vi "Average Sectors.vi"   [LabVIEW 2013]
uses:
  Globals/Accumulated Sector Intensity.vi
  Globals/Sector Parameter Global.vi
  <vilib>/rvi/Memory/Memory_Emulation/nirvimemoryFastEmulationFpgaImpl.vi
  <instcachedir>/0/nirvimemoryFastEmulationFpgaImpl_5FBAB50466BC4C939F684F8805638BFC.lvgen/nirvimemoryFastEmulationFpgaImpl_5FBAB50466BC4C939F684F8805638BFC_006.vi
  <vilib>/rvi/DataTransferAndStorage/Container/Common/niFpgaContainerGetUniqueNameForEmu.vi
  <vilib>/rvi/Memory/Memory_Emulation/nirvimemoryFastEmulation.vi
  <vilib>/rvi/Memory/Memory_Emulation/nirvimemoryEmulation.vi
  <vilib>/rvi/FIFO/Fifo_Resource/nirvififoEmulationWriteFpgaImpl.vi
  <vilib>/rvi/DataTransferAndStorage/Container/XNode/niFpgaContainer.xnode
  <vilib>/rvi/FIFO/Fifo_Resource/nirvififoEmulationWrite.vi
types:
  T1 = cluster{"Accumulated Intensity":u32, "Count":u16}
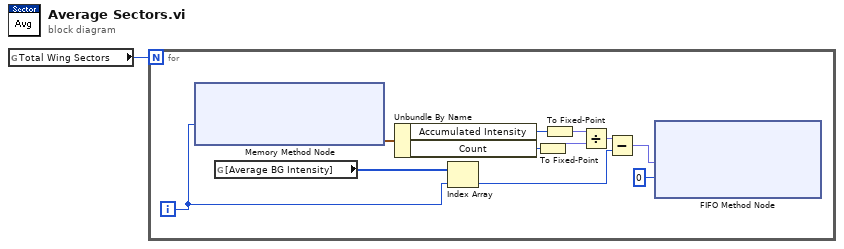
[diagram p0: block diagram]
diagram:
  n1 = global read "Accumulated Sector Intensity.vi" "Total Wing Sectors"() -> (w1:u8)
  n2 = for {
    N: w1 -> [_]
    i -> [w5]
    n3 = xnode ("Memory Method Node")("Address"=w5) -> ("Data"=w8:T1)  [unwired: 1 in, 1 out]
    n4 = global read "Sector Parameter Global.vi" "[Average BG Intensity]"() -> (w6:u8[])
    n5 = Unbundle By Name(w8) -> ("Accumulated Intensity"=w12:u32, "Count"=w11:u16)
    n6 = Index Array(array=w6, index=w5) -> (element=w3:u8)
    n7 = To Fixed-Point(number=w11) -> (fixed-point=w9:fxp<+,16,16>)  [unwired: 1 in]
    n8 = To Fixed-Point(number=w12) -> (fixed-point=w10:fxp<+,32,32>)  [unwired: 1 in]
    n9 = Divide(x=w10, y=w9) -> (x/y=w4:fxp<+,8,8>)
    n10 = Subtract(x=w4, y=w3) -> (x-y=w2:fxp<+/-,9,9>)
    n11 = xnode ("FIFO Method Node")("Element"=w2, "Timeout"=0) -> ()  [unwired: 1 in, 2 out]
  }
